vi "YAML Get Field Value Double.vi"(10 "field name":string, 11 "array of strings":string[][](array[string])) -> (3 "Numeric Control":dbl)   [LabVIEW 2011]
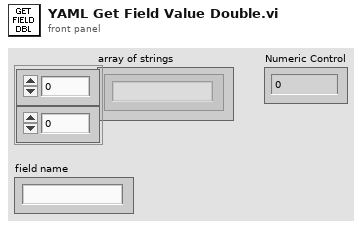
[diagram p1: front panel]
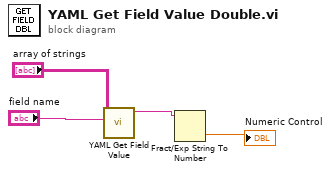
[diagram p0: block diagram]
diagram:
  n1 = call "YAML Get Field Value.vi"("field name"="field name", "array of strings"="array of strings") -> ("field value"=w2:string)  [unwired: 9 in]
  n2 = Fract/Exp String To Number(string=w2) -> (number=→"Numeric Control":dbl)  [unwired: 3 in, 1 out]
